vi "calcularVref.vi"(8 "error in (no error)":errorcluster, 11 "Prueba10 in":refnum<class "Prueba10.lvclass">) -> (0 "error out":errorcluster, 3 "Prueba10 out":refnum<class "Prueba10.lvclass">)   [LabVIEW 2019, in "Prueba10.lvclass"]
uses:
  Prueba10.lvclass
  Prueba10.lvclass/Prueba10.ctl
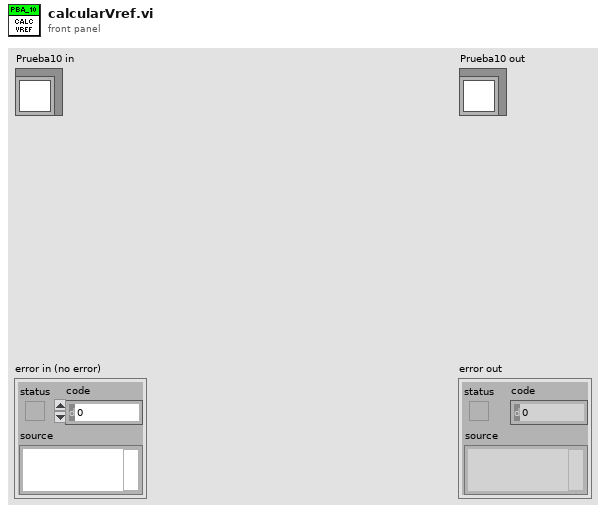
[diagram p1: front panel]
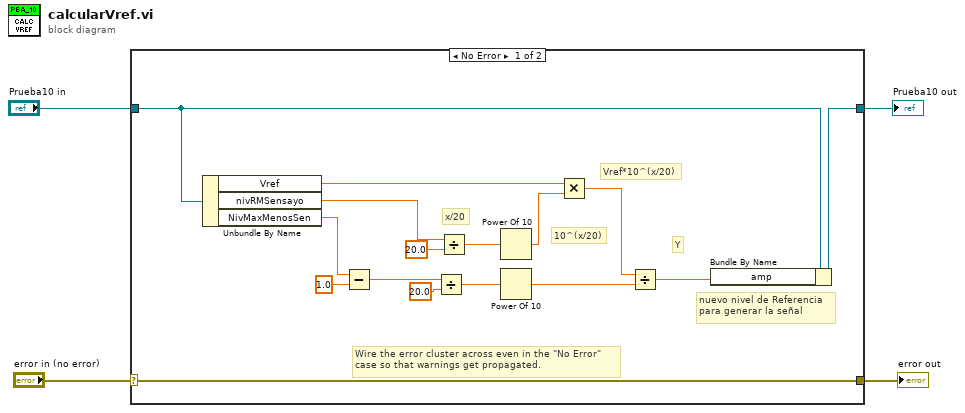
[diagram p0: block diagram]
diagram:
  n1 = case shown="No Error" "error in (no error)" {
    selector: "error in (no error)" -> [w20 w22]
    tunnel: [w20 w22] -> w3
    tunnel: [w6 w21] -> w1
    tunnel: "Prueba10 in" -> [w19 w21]
    frame No Error {
      # "Y"
      # "nuevo nivel de Referencia\npara generar la señal"
      # "Vref*10^(x/20)"
      # "10^(x/20)"
      # "x/20"
      # "Wire the error cluster across even in the \"No Error\"\ncase so that warnings get propagated."
      n2 = Unbundle By Name(w19) -> ("Vref"=w18:dbl, "nivRMSensayo"=w17:dbl, "NivMaxMenosSen"=w11:dbl)
      n3 = Subtract(x=w11, y=1.0) -> (x-y=w9:dbl)
      n4 = Divide(x=w9, y=20.0) -> (x/y=w8:dbl)
      n5 = Divide(x=w17, y=20.0) -> (x/y=w15:dbl)
      n6 = Power Of 10(x=w15) -> (10^x=w14:dbl)
      n7 = Power Of 10(x=w8) -> (10^x=w7:dbl)
      n8 = Multiply(x=w18, y=w14) -> (x*y=w13:dbl)
      n9 = Divide(x=w13, y=w7) -> (x/y=w5:dbl)
      n10 = Bundle By Name(cluster=w19, "amp"=w5) -> (w6:refnum<class "Prueba10.lvclass">)
    }
    frame Error {
    }
  }
  "error out" <- w3
  "Prueba10 out" <- w1
